vi "InitializeTrigger.vi"(8 "error in (no error)":errorcluster, 11 "Highland T564 DDG in":refnum<class "Highland T564 DDG.lvclass">) -> (0 "error out":errorcluster, 3 "Highland T564 DDG out":refnum<class "Highland T564 DDG.lvclass">)   [LabVIEW 2020, in "Highland T564 DDG.lvclass"]
doc: "Initialize the physical device trigger"
uses:
  Highland T564 DDG.lvclass
  SupportLibraries/DeviceSpecific/HighlandT560Lib/T560TriggerClass/T560Trigger.lvclass
  C:/GEECS/Developers Version/source/Device Drivers/Highland T564 DDG/SupportLibraries/DeviceSpecific/HighlandT560Lib/T560ChannelClass/T560Channel.lvclass
  SupportLibraries/DeviceSpecific/HighlandT560Lib/Common/TypeDefs/ChannelName.ctl
  Highland T564 DDG.lvclass/Highland T564 DDG.ctl
  SupportLibraries/DeviceSpecific/HighlandT560Lib/T560SessionClass/T560Session.lvclass
  SupportLibraries/DeviceSpecific/HighlandT560Lib/T560ChannelClass/T560Channel.lvclass
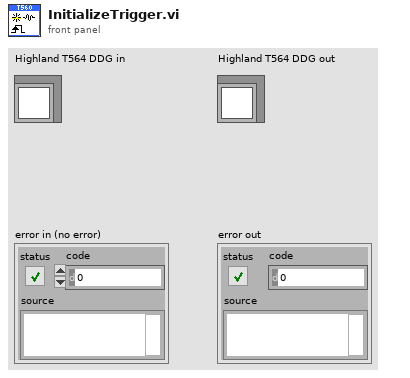
[diagram p1: front panel]
types:
  T1 = typedef "T560Channel.lvclass/ChannelName.ctl" = enum16{"Null", "A", "B", "C", "D", "Trigger"}
  T2 = typedef "TriggerImpedance.ctl" = enum16{"10KOhm", "50Ohms"}
  T3 = typedef "TriggerSource.ctl" = enum16{"Rising", "Falling", "Internal 80MHz", "Internal DDS", "Remote", "Disabled"}
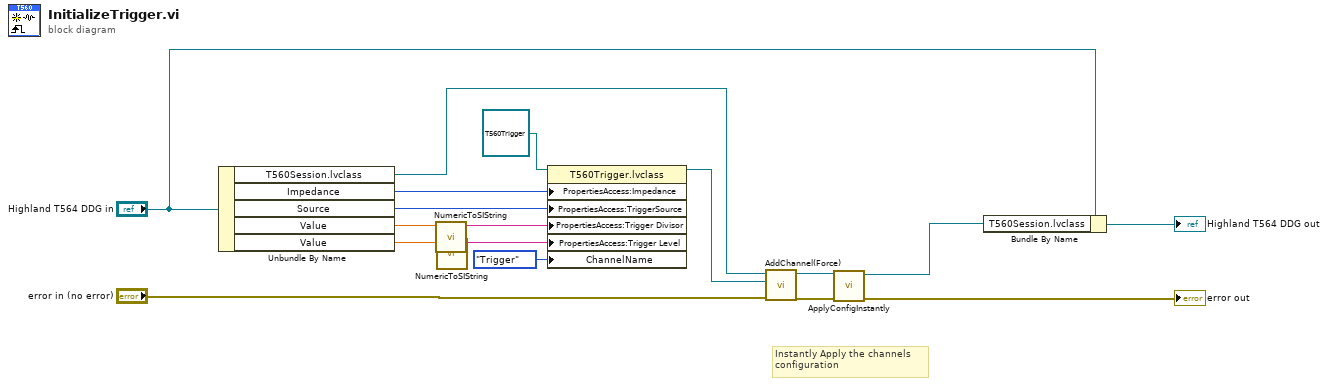
[diagram p0: block diagram]
diagram:
  # "Instantly Apply the channels \nconfiguration"
  n1 = Unbundle By Name("Highland T564 DDG in") -> ("T560Session.lvclass"=w1:refnum<class "T560Session.lvclass">, "Impedance"=w13:T2, "Source"=w12:T3, "Value"=w11:dbl, "Value"=w9:dbl)
  n2 = call "NumericToSIString.vi"("Numeric"=w11) -> ("SI_String"=w10:string)  [unwired: 9 in, 1 out]
  n3 = call "NumericToSIString.vi"("Numeric"=w9) -> ("SI_String"=w8:string)  [unwired: 9 in, 1 out]
  n4 = property class="T560Trigger.lvclass"(reference=refnum<class "T560Trigger.lvclass"> refnum ("Highlandt564.lvlib:T560Trigger.lvclass"), "PropertiesAccess:Impedance"=w13, "PropertiesAccess:TriggerSource"=w12, "PropertiesAccess:Trigger Divisor"=w10, "PropertiesAccess:Trigger Level"=w8, "ChannelName"=ChannelName."Trigger") -> (reference out=w7:refnum<class "T560Trigger.lvclass">)  [unwired: 1 in, 1 out]
  n5 = call-dynamic "AddChannel(Force).vi"("error in (no error)"="error in (no error)", "T560Channel.lvclass"=w7, "T560Session in"=w1) -> ("error out"=w4:errorcluster, "T560Session out"=w6:refnum<class "T560Session.lvclass">)  [unwired: 7 in]
  n6 = call-dynamic "ApplyConfigInstantly.vi"("error in"=w4, "T560Session in"=w6) -> ("error out"=→"error out":errorcluster, "T560Session out"=w5:refnum<class "T560Session.lvclass">)  [unwired: 8 in]
  n7 = Bundle By Name(cluster="Highland T564 DDG in", "T560Session.lvclass"=w5) -> (→"Highland T564 DDG out":refnum<class "Highland T564 DDG.lvclass">)
